vi "V Hopper Initialization.vi"() -> (0 "V Hopper Ref 2":T1, 3 "V Hopper Ref 1":T1)   [LabVIEW 2025]
uses:
  <vilib>/Rock Robotics/WPI/MotorControl/WPI_MotorControlDeviceRef.ctl
  <vilib>/Rock Robotics/WPI/MotorControl/WPI_MotorControlType.ctl
  <vilib>/Rock Robotics/SystemInterfaces/DIO/FPGA_DIOPWMChannel.ctl
  <vilib>/Rock Robotics/WPI/PWM/WPI_PWMDeadband.ctl
  <vilib>/Rock Robotics/SystemInterfaces/DIO/FPGA_DIOChannel.ctl
  <vilib>/Rock Robotics/WPI/ThirdParty/REV Robotics/REVLib/Typedef/Spark MAX Idle Mode.ctl
  <vilib>/Rock Robotics/WPI/ThirdParty/REV Robotics/REVLib/SubVI/Public/SPARK Open Brushless.vi
  <vilib>/Rock Robotics/WPI/ThirdParty/REV Robotics/REVLib/SubVI/Public/SPARK Configure Basic Idle Mode.vi
  <vilib>/Rock Robotics/WPI/ThirdParty/REV Robotics/REVLib/SubVI/Public/SPARK Configure Soft Limit Forward.vi
  <vilib>/Rock Robotics/WPI/ThirdParty/REV Robotics/REVLib/SubVI/Public/SPARK Configure Soft Limit Reverse.vi
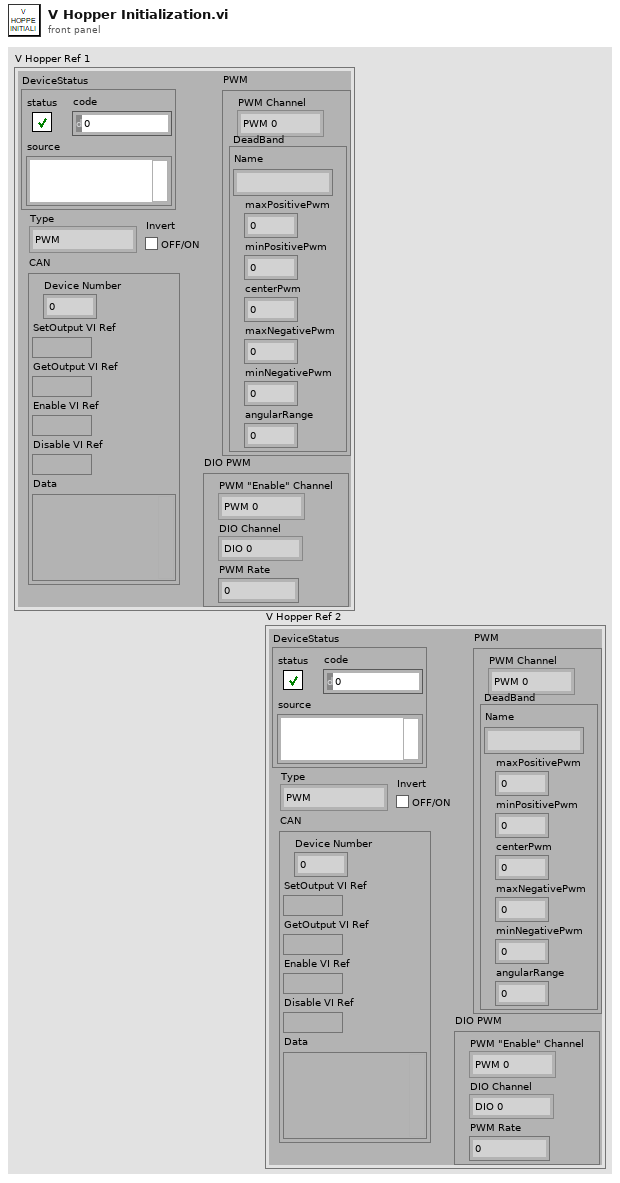
[diagram p1: front panel]
types:
  T1 = typedef "WPI_MotorControlDeviceRef.ctl" = cluster{"DeviceStatus":errorcluster, "Type":T2, "PWM":cluster{"PWM Channel":T3, "DeadBand":T4}, "CAN":cluster{"Device Number":u8, "SetOutput VI Ref":variant, "GetOutput VI Ref":variant, "Enable VI Ref":variant, "Disable VI Ref":variant, "Data":variant}, "Invert":bool, "DIO PWM":cluster{"PWM \"Enable\" Channel":T3, "DIOChannel":T5, "PWM Rate":dbl}}
  T2 = typedef "WPI_MotorControlType.ctl" = enum16{"PWM", "CAN", "DIO PWM"}
  T3 = typedef "FPGA_DIOPWMChannel.ctl" = enum8{"PWM 0", "PWM 1", "PWM 2", "PWM 3", "PWM 4", "PWM 5", "PWM 6", "PWM 7", "PWM 8", "PWM 9", "PWM MXP 0", "PWM MXP 1", "PWM MXP 2", "PWM MXP 3", "PWM MXP 4", "PWM MXP 5", "PWM MXP 6", "PWM MXP 7", "PWM MXP 8", "PWM MXP 9", "Invalid"}
  T4 = typedef "WPI_PWMDeadband.ctl" = cluster{"Name":string, "maxPositivePwm":i32, "minPositivePwm":i32, "centerPwm":i32, "maxNegativePwm":i32, "minNegativePwm":i32, "angularRange":u16}
  T5 = typedef "FPGA_DIOChannel.ctl" = enum8{"DIO 0", "DIO 1", "DIO 2", "DIO 3", "DIO 4", "DIO 5", "DIO 6", "DIO 7", "DIO 8", "DIO 9", "DIO MXP 0", "DIO MXP 1", "DIO MXP 2", "DIO MXP 3", "DIO MXP 4", "DIO MXP 5", "DIO MXP 6", "DIO MXP 7", "DIO MXP 8", "DIO MXP 9", "DIO MXP 10", "DIO MXP 11", "DIO MXP 12", "DIO MXP 13", "DIO MXP 14", "DIO MXP 15", "SPI Port CS1", "SPI Port CS2", "SPI Port CS3", "SPI Port MISO", "SPI Port MOSI", "Invalid"}
  T6 = typedef "Spark MAX Idle Mode.ctl" = enum16{"Coast", "Brake"}
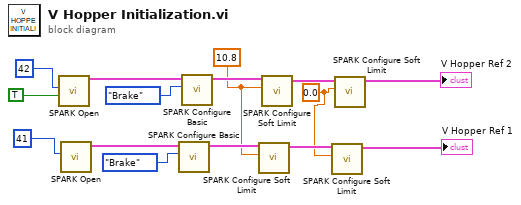
[diagram p0: block diagram]
diagram:
  w3 = 0.0 ("Soft Limit")
  w8 = 10.8 ("Soft Limit")
  n1 = call-poly <vilib>:"SPARK Open.vi"("Invert"=TRUE, "Device Number"=u8 42) -> ("MotorControlDeviceRef"=w7:T1)  [unwired: 8 in, 1 out]
  n2 = call-poly <vilib>:"SPARK Open.vi"("Device Number"=u8 41) -> ("MotorControlDeviceRef"=w11:T1)  [unwired: 9 in, 1 out]
  n3 = call-poly <vilib>:"SPARK Configure Basic.vi"("Idle Mode"=Spark_MAX_Idle_Mode."Brake", "MotorControlDeviceRef in"=w11) -> ("MotorControlDeviceRef out"=w13:T1)  [unwired: 8 in, 1 out]
  n4 = call-poly <vilib>:"SPARK Configure Basic.vi"("Idle Mode"=Spark_MAX_Idle_Mode."Brake", "MotorControlDeviceRef in"=w7) -> ("MotorControlDeviceRef out"=w10:T1)  [unwired: 8 in, 1 out]
  n5 = call-poly <vilib>:"SPARK Configure Soft Limit.vi"("Soft Limit"=w8, "MotorControlDeviceRef in"=w13) -> ("MotorControlDeviceRef out"=w5:T1)  [unwired: 8 in, 1 out]
  n6 = call-poly <vilib>:"SPARK Configure Soft Limit.vi"("Soft Limit"=w8, "MotorControlDeviceRef in"=w10) -> ("MotorControlDeviceRef out"=w4:T1)  [unwired: 8 in, 1 out]
  n7 = call-poly <vilib>:"SPARK Configure Soft Limit.vi"("Soft Limit"=w3, "MotorControlDeviceRef in"=w5) -> ("MotorControlDeviceRef out"=→"V Hopper Ref 1":T1)  [unwired: 8 in, 1 out]
  n8 = call-poly <vilib>:"SPARK Configure Soft Limit.vi"("Soft Limit"=w3, "MotorControlDeviceRef in"=w4) -> ("MotorControlDeviceRef out"=→"V Hopper Ref 2":T1)  [unwired: 8 in, 1 out]
